vi "Init.vi"(8 "error in (no error)":errorcluster, 11 "Pic Json Generator in":refnum<class "Pic Json Generator.lvclass">) -> (0 "error out":errorcluster, 3 "Pic Json Generator out":refnum<class "Pic Json Generator.lvclass">)   [LabVIEW 2018, in "Pic Json Generator.lvlib" / "Pic Json Generator.lvclass"]
uses:
  Pic Json Generator.lvclass
  Pic Json Generator.lvclass/Pic Json Generator.ctl
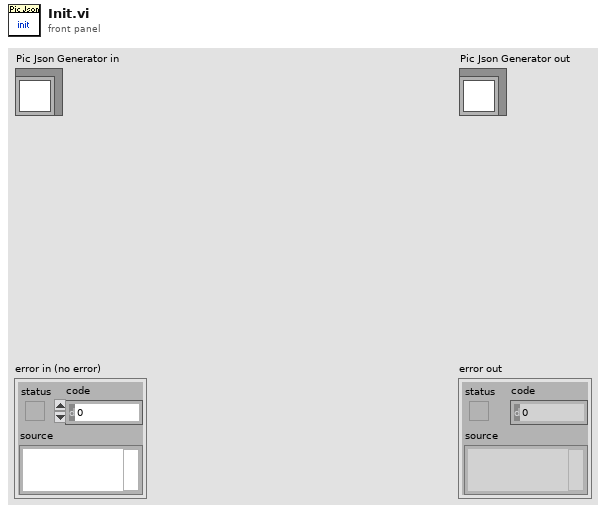
[diagram p1: front panel]
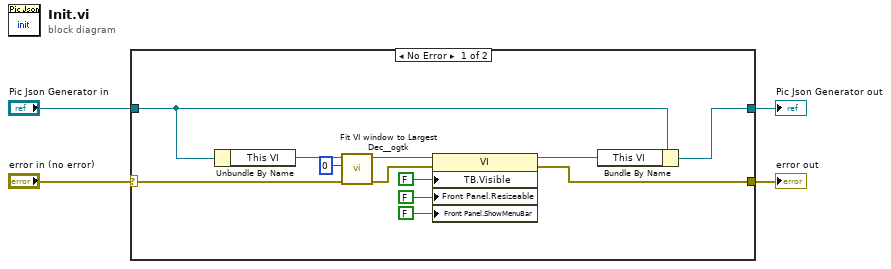
[diagram p0: block diagram]
diagram:
  n1 = case shown="No Error" "error in (no error)" {
    selector: "error in (no error)" -> [w8 w18]
    tunnel: [w7 w18] -> w3
    tunnel: [w6 w17] -> w1
    tunnel: "Pic Json Generator in" -> [w9 w17]
    frame No Error {
      n2 = Unbundle By Name(w9) -> ("This VI"=w16:refnum<vi>)
      n3 = call <userlib>:"Fit VI window to Largest Dec__ogtk.vi"("error in (no error)"=w8, "border spacing (2 px)"=0, "VI Ref (calling VI)"=w16) -> ("error out"=w11:errorcluster, "dup VI Ref"=w14:refnum<vi>)  [unwired: 3 in]
      n4 = property class="VI"(reference=w14, error in=w11, "TB.Visible"=FALSE ("Tool Bar:Visible"), "Front Panel.Resizeable"=FALSE ("Front Panel Window:Resizable"), "Front Panel.ShowMenuBar"=FALSE ("Front Panel Window:Resizable")) -> (reference out=w10:refnum<vi>, error out=w7:errorcluster)
      n5 = Bundle By Name(cluster=w9, "This VI"=w10) -> (w6:refnum<class "Pic Json Generator.lvclass">)
    }
    frame Error {
    }
  }
  "error out" <- w3
  "Pic Json Generator out" <- w1
